vi "Recursive Add Tag.vi"(8 "error in (no error)":errorcluster, 9 "Child Text":string[](array[string]), 10 "Tag":string, 11 "Tag Tree In":refnum<class "Tag Tree.lvclass">) -> (0 "error out":errorcluster, 3 "Tag Tree Out":refnum<class "Tag Tree.lvclass">)   [LabVIEW 2020, in "Tree Helpers.lvlib" / "Tag Tree.lvclass"]
uses:
  Tag Tree.lvclass
  Tag Tree.lvclass/Tag Tree.ctl
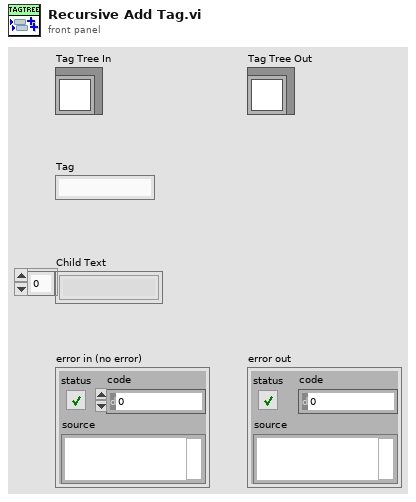
[diagram p1: front panel]
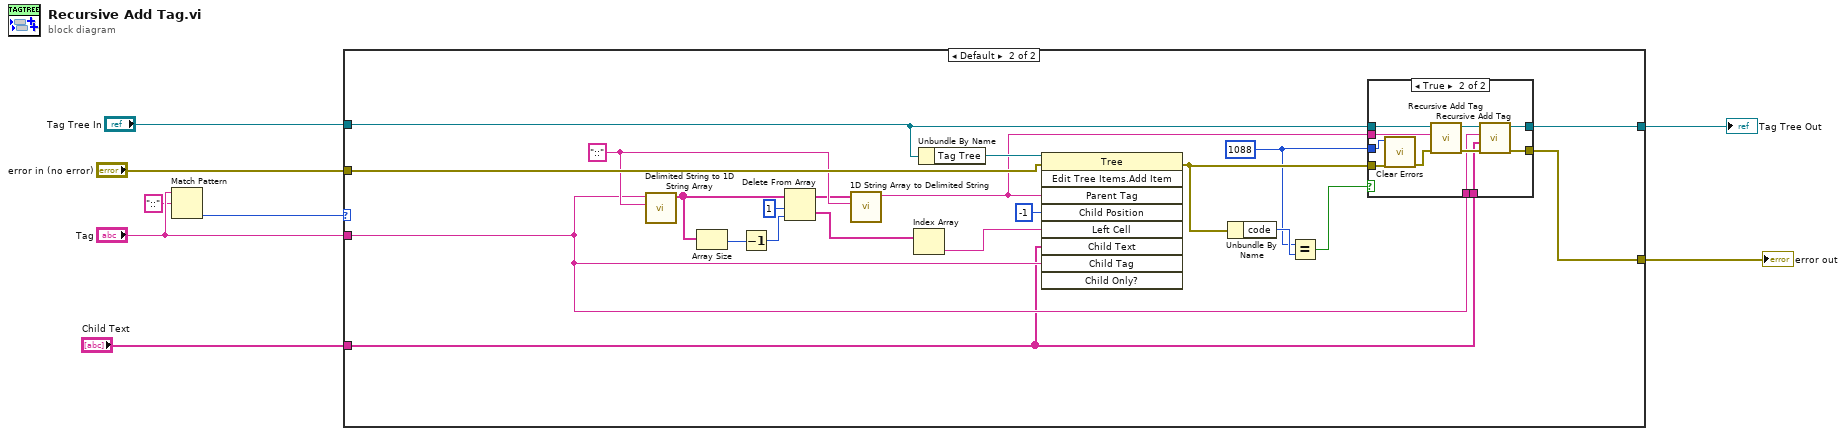
[diagram p0: block diagram]
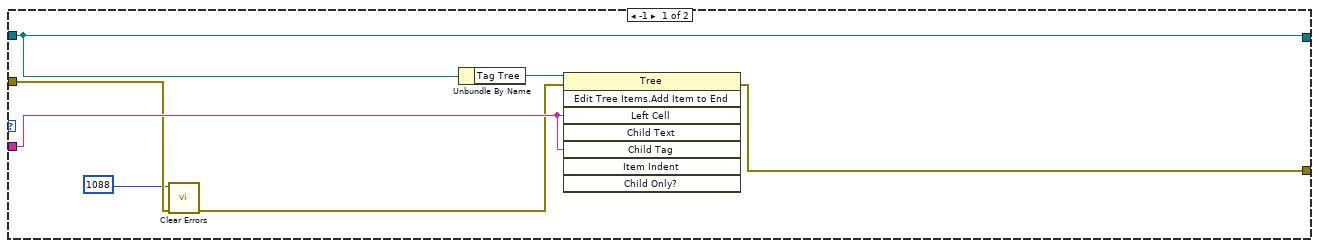
[diagram p2: hidden frame]
diagram:
  n1 = Match Pattern(string="Tag", regular expression="::") -> (offset past match=w2:i32)  [unwired: 1 in, 3 out]
  n2 = case shown="Default" w2 {
    tunnel: "error in (no error)" -> [w11 w36]
    tunnel: [w13 w24] -> w7
    tunnel: "Tag Tree In" -> [w14 w23]
    tunnel: [w14 w22] -> w5
    tunnel: "Tag" -> [w12 w19]
    tunnel: "Child Text" -> [_ w17]
    frame -1 {
      n3 = call <vilib>:"Clear Errors.vi"("error in (no error)"=w11, "specific error code to clear (0: all)"=1088) -> ("error out"=w9:errorcluster)  [unwired: 4 in, 1 out]
      n4 = Unbundle By Name(w14) -> ("Tag Tree"=w15:refnum<vi>)
      n5 = invoke class="Tree" method="Edit Tree Items.Add Item to End"(reference=w15, error in=w9, "Left Cell"=w12, "Child Tag"=w12) -> (error out=w13:errorcluster)  [unwired: 4 in, 7 out]
    }
    frame Default {
      w16 = 1088
      w31 = "::" ("delimiter")
      n6 = call <vilib>:"Delimited String to 1D String Array.vi"("delimiter"=w31, "delimited string"=w19) -> ("string array"=w28:string[])  [unwired: 9 in]
      n7 = Array Size(array=w28) -> (size(s)=w26:i32)
      n8 = Decrement(x=w26) -> (x-1=w27:i32)
      n9 = Delete From Array(array=w28, length=1, index=w27) -> (deleted portion=w33:string[], array with subset deleted=w30:string[])
      n10 = call <vilib>:"1D String Array to Delimited String.vi"("delimiter"=w31, "string array"=w30) -> ("delimited string"=w21:string)  [unwired: 9 in]
      n11 = Index Array(array=w33) -> (element=w34:string)  [unwired: 1 in]
      n12 = Unbundle By Name(w23) -> ("Tag Tree"=w32:refnum<vi>)
      n13 = invoke class="Tree" method="Edit Tree Items.Add Item"(reference=w32, error in=w36, "Parent Tag"=w21, "Child Position"=-1, "Left Cell"=w34, "Child Text"=w17, "Child Tag"=w19) -> (error out=w25:errorcluster)  [unwired: 2 in, 8 out]
      n14 = Unbundle By Name(w25) -> ("code"=w35:i32)
      n15 = Equal?(x=w16, y=w35) -> (x = y?=w20:bool)
      n16 = case shown="True" w20 {
        tunnel: w25 -> [w37 w41]
        tunnel: [w37 w44] -> w24
        tunnel: w23 -> [w38 w49]
        tunnel: [w38 w46] -> w22
        tunnel: w21 -> [_ w48]
        tunnel: w19 -> [_ w43]
        tunnel: w17 -> [_ w42]
        tunnel: w16 -> [_ w40]
        frame False {
        }
        frame True {
          n17 = call <vilib>:"Clear Errors.vi"("error in (no error)"=w41, "specific error code to clear (0: all)"=w40) -> ("error out"=w39:errorcluster)  [unwired: 4 in, 1 out]
          n18 = call "Recursive Add Tag.vi"("error in (no error)"=w39, "Tag"=w48, "Tag Tree In"=w49) -> ("error out"=w45:errorcluster, "Tag Tree Out"=w47:refnum<class "Tag Tree.lvclass">)  [unwired: 7 in]
          n19 = call "Recursive Add Tag.vi"("error in (no error)"=w45, "Child Text"=w42, "Tag"=w43, "Tag Tree In"=w47) -> ("error out"=w44:errorcluster, "Tag Tree Out"=w46:refnum<class "Tag Tree.lvclass">)  [unwired: 6 in]
        }
      }
    }
  }
  "error out" <- w7
  "Tag Tree Out" <- w5
